vi "Global.vi"() -> ()   [LabVIEW 2020]
panel:
  out "芯轴码":string
  out "工位二扭矩":dbl
  out "工位一扭矩":dbl
  in  "可信度范围":T1
  in  "可信度检测引用句柄":refnum<vi>
  in  "工位":enum16{"左工位", "右工位"}(ring)
  out "SROC 2":i32
  out "PROC 2":i32
  out "T2ROC_1+T2ROC_2 2":i32
  out "T1ROC_1+T1ROC_2 2":i32
  out "T2ROC_1 2":i32
  out "T1ROC_1 2":i32
  out "产品型号":string
  out "工位二S":dbl
  out "工位二P":dbl
  in  "保护角度":dbl
  in  "跳过优化":bool
  in  "8点复测":bool
  in  "动态优化复测":bool
  in  "动态优化判定":T2
  in  "动态优化完成":bool
  in  "静态标定判定":T3
  out "动态优化参数":dbl[](array[numeric])
  out "T1":dbl
  out "T2均值":dbl
  out "T1均值":dbl
  out "Sxinhao":dbl[](array[numeric])
  out "Pxinhao":dbl[](array[numeric])
  out "子数组 2":dbl[](array[numeric])
  out "子数组":dbl[](array[numeric])
  out "T2ROC3":i32
  out "T1ROC3":i32
  out "VRes":dbl
  out "PROC_1":i32
  out "T2ROC1+2+3":i32
  out "T1ROC1+2+3":i32
  out "Vresccw_min":dbl
  out "Vrescw_min":dbl
  out "SROC":i32
  out "PROC":i32
  out "T2ROC_1+T2ROC_2":i32
  out "T1ROC_1+T1ROC_2":i32
  out "T2ROC_1":i32
  out "T1ROC_1":i32
  out "工位一S":dbl
  out "工位一P":dbl
  in  "P/S采集":bool
  in  "方向":bool
  in  "动态优化引用句柄":refnum<vi>
  in  "联机模式":enum16{"单机", "追溯"}(ring)=enum."追溯"
  out "用户信息":T4
  in  "复检判定参数":T5
  out "工位二扭矩偏移":cluster{"正向":dbl, "逆向":dbl}
  out "工位一扭矩偏移":cluster{"正向":dbl, "逆向":dbl}
  out "复检参数":T6
  out "扭矩":cluster{"工位一":dbl, "工位二":dbl}
  out "工位二T2":dbl
  out "工位二T1":dbl
  out "工位一T2":dbl
  out "工位一T1":dbl
  in  "工位占空比采集":bool
  in  "传感器特性用句柄":refnum<vi>
  in  "程序固化引用句柄":refnum<vi>
  in  "静态标定引用句柄":refnum<vi>
  out "S7 Link":refnum<k5>
  out "产品编号":string
  in  "计时开始":bool
  in  "计时复位":bool
  in  "IO_Stop":bool
  in  "合格数量":i32
  in  "生产数量":i32
  in  "试验项目":bool[](array[boolean])
  out "模式":u32
  in  "更换产品":refnum<vi>
  in  "提示信息":refnum<vi>
  in  "程序自动":refnum<vi>
  in  "报警图标":refnum<vi>
  in  "程序关闭":bool
  in  "Info":refnum<vi>
  in  "Result":refnum<vi>
  in  "批次":refnum<vi>
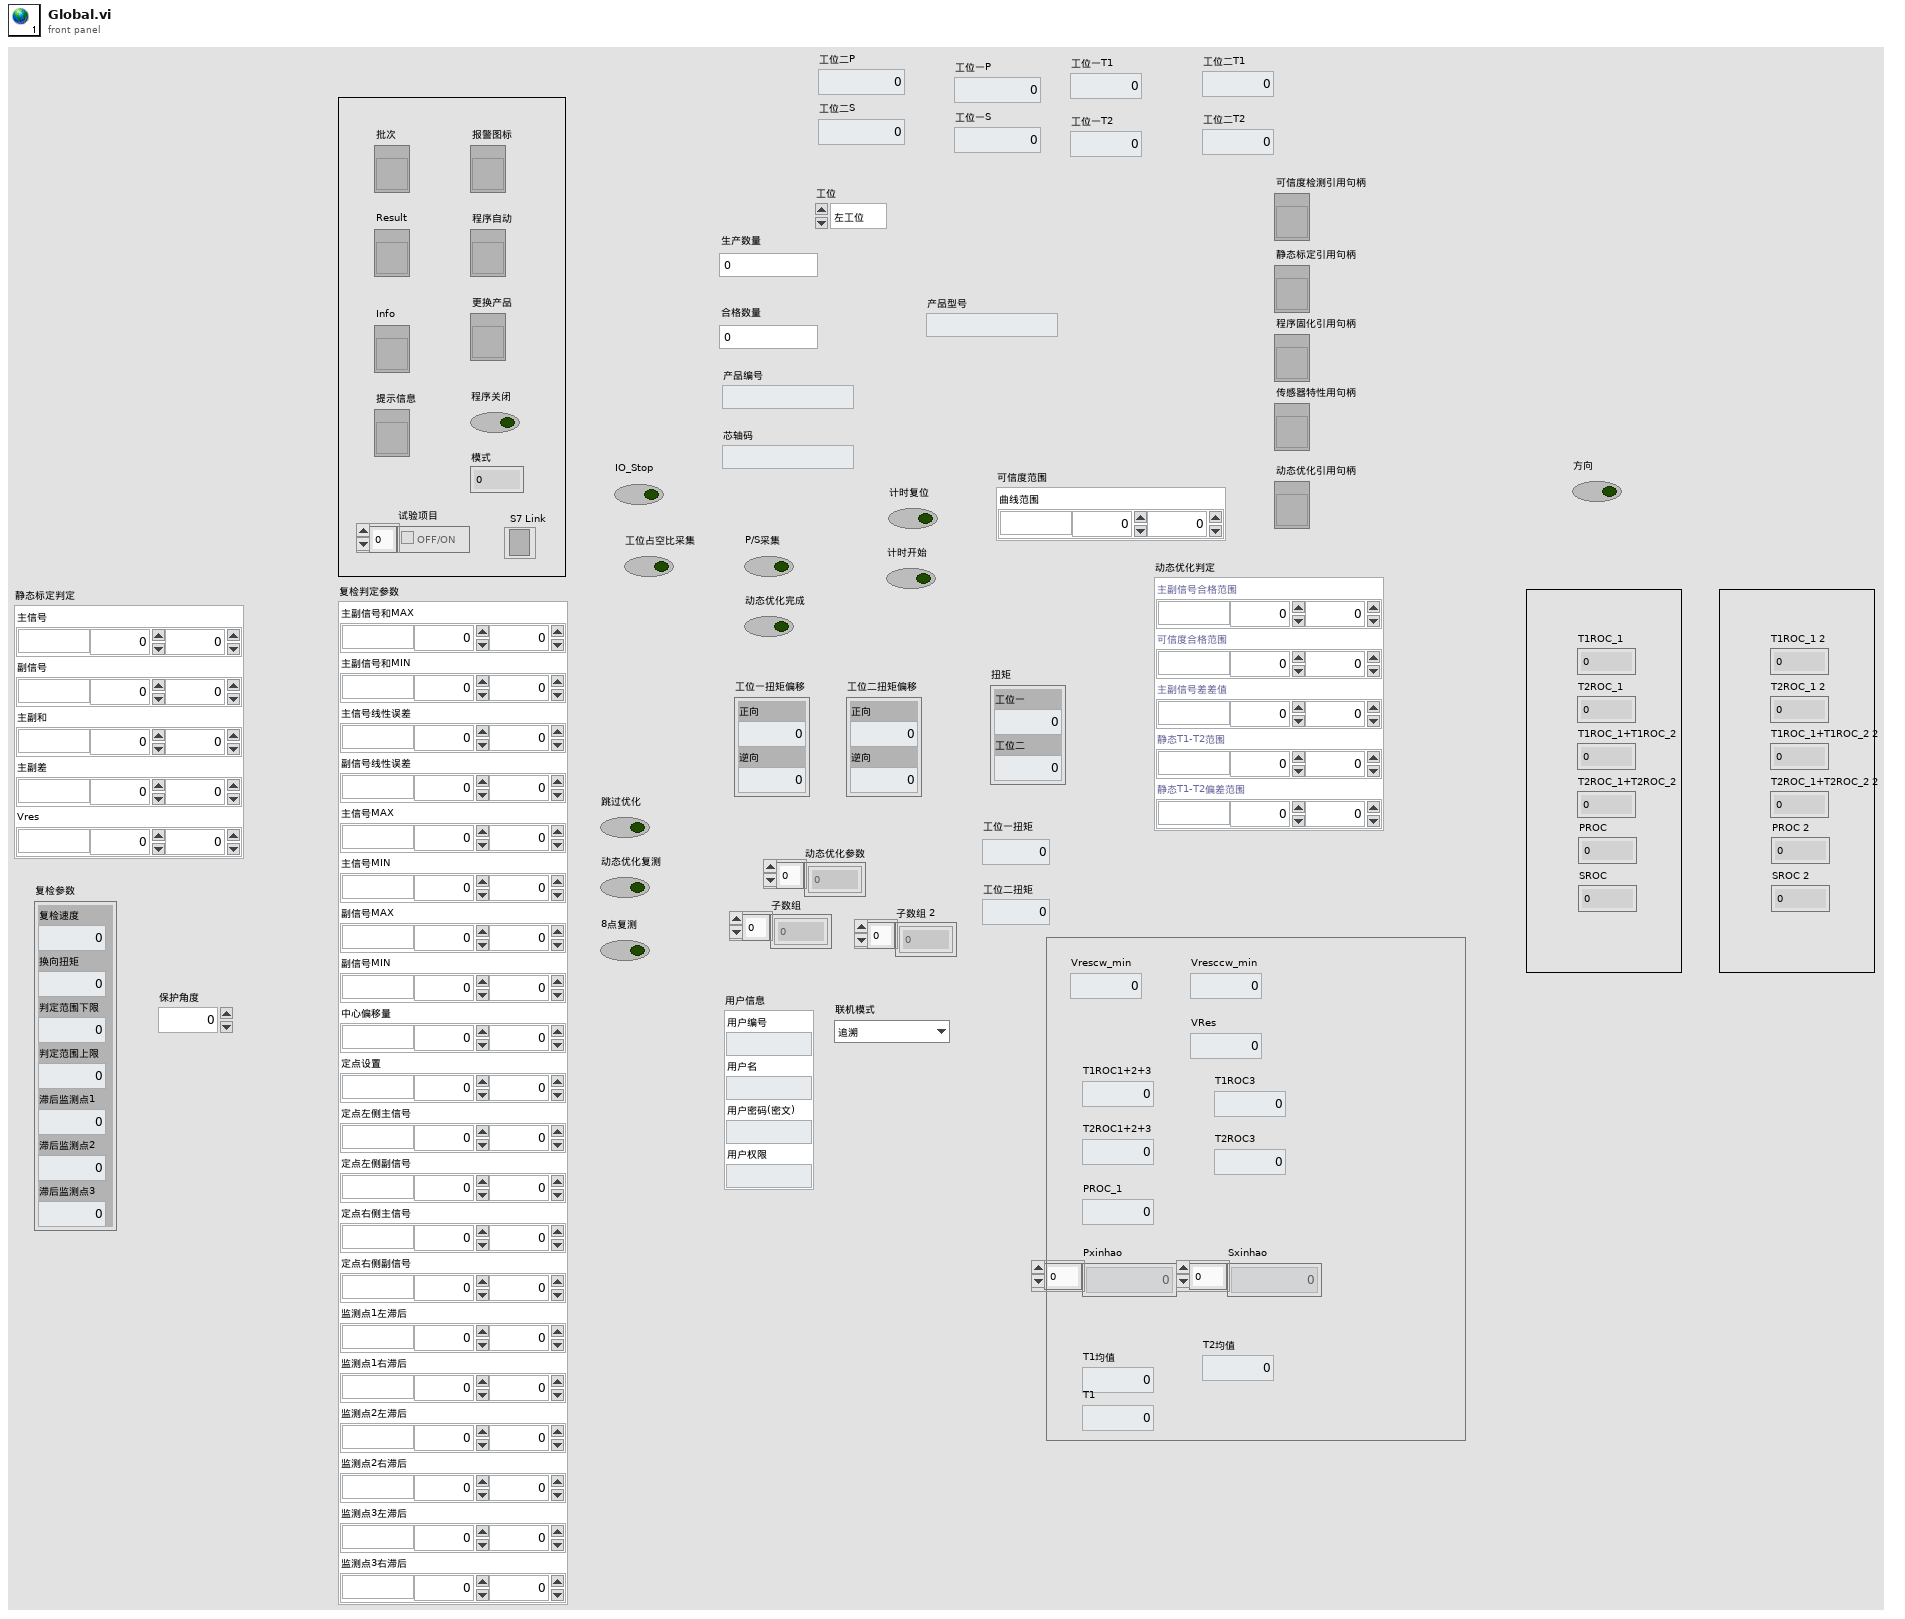
[diagram p1: front panel]
types:
  T1 = cluster{"曲线范围":cluster{"单位":string, "角度下限":dbl, "角度上限":dbl}}
  T2 = cluster{"主副信号合格范围":cluster{"单位":string, "下限":dbl, "上限":dbl}, "可信度合格范围":cluster{"单位":string, "下限":dbl, "上限":dbl}, "主副信号差差值":cluster{"单位":string, "下限":dbl, "上限":dbl}, "静态T1-T2范围":cluster{"单位":string, "下限":dbl, "上限":dbl}, "静态T1-T2偏差范围":cluster{"单位":string, "下限":dbl, "上限":dbl}}
  T3 = cluster{"主信号":cluster{"单位":string, "下限":dbl, "上限":dbl}, "副信号":cluster{"单位":string, "下限":dbl, "上限":dbl}, "主副和":cluster{"单位":string, "下限":dbl, "上限":dbl}, "主副差":cluster{"单位":string, "下限":dbl, "上限":dbl}, "Vres":cluster{"单位":string, "下限":dbl, "上限":dbl}}
  T4 = cluster{"用户编号":string, "用户名":string, "用户密码(密文)":string, "用户权限":string}
  T5 = cluster{"主副信号和MAX":cluster{"单位":string, "下限":dbl, "上限":dbl}, "主副信号和MIN":cluster{"单位":string, "下限":dbl, "上限":dbl}, "主信号线性误差":cluster{"单位":string, "下限":dbl, "上限":dbl}, "副信号线性误差":cluster{"单位":string, "下限":dbl, "上限":dbl}, "主信号MAX":cluster{"单位":string, "下限":dbl, "上限":dbl}, "主信号MIN":cluster{"单位":string, "下限":dbl, "上限":dbl}, "副信号MAX":cluster{"单位":string, "下限":dbl, "上限":dbl}, "副信号MIN":cluster{"单位":string, "下限":dbl, "上限":dbl}, "中心偏移量":cluster{"单位":string, "下限":dbl, "上限":dbl}, "定点设置":cluster{"单位":string, "下限":dbl, "上限":dbl}, "定点左侧主信号":cluster{"单位":string, "下限":dbl, "上限":dbl}, "定点左侧副信号":cluster{"单位":string, "下限":dbl, "上限":dbl}, "定点右侧主信号":cluster{"单位":string, "下限":dbl, "上限":dbl}, "定点右侧副信号":cluster{"单位":string, "下限":dbl, "上限":dbl}, "监测点1左滞后":cluster{"单位":string, "下限":dbl, "上限":dbl}, "监测点1右滞后":cluster{"单位":string, "下限":dbl, "上限":dbl}, "监测点2左滞后":cluster{"单位":string, "下限":dbl, "上限":dbl}, "监测点2右滞后":cluster{"单位":string, "下限":dbl, "上限":dbl}, "监测点3左滞后":cluster{"单位":string, "下限":dbl, "上限":dbl}, "监测点3右滞后":cluster{"单位":string, "下限":dbl, "上限":dbl}}
  T6 = cluster{"复检速度":dbl, "换向扭矩":dbl, "判定范围下限":dbl, "判定范围上限":dbl, "滞后监测点1":dbl, "滞后监测点2":dbl, "滞后监测点3":dbl}
diagram:
